vi "add.test.vi"() -> ()   [LabVIEW 2016]
uses:
  <vilib>/addons/_JKI Toolkits/Caraya/classes/Assert/Assert Equal Value_Variant.vi
  <vilib>/addons/_JKI Toolkits/Caraya/classes/Test/Test.lvclass
  <vilib>/addons/_JKI Toolkits/Caraya/classes/Assert/Assert.lvclass
panel:
  out "error out":errorcluster
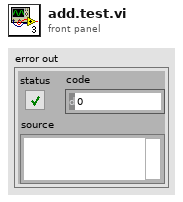
[diagram p1: front panel]
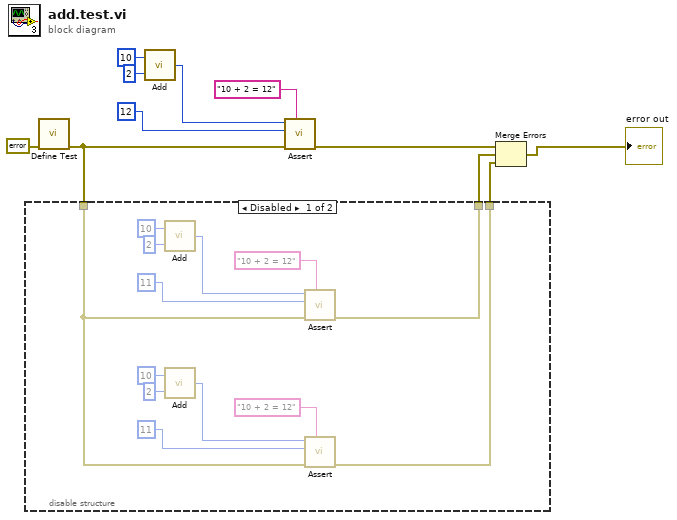
[diagram p0: block diagram]
diagram:
  n1 = call <vilib>:"Define Test.vi"("error in (no error)"=errorcluster {"status"=FALSE, "code"=0, "source"=""}) -> ("error out"=w2:errorcluster)  [unwired: 10 in]
  n2 = disable-structure shown="Disabled" {
    disable-tunnel: [w14 _] -> w3
    disable-tunnel: w2 -> [w13 _]
    disable-tunnel: [w12 _] -> w1
    frame Disabled {
      n3 = call "Add.vi"("y"=2, "x"=10) -> ("x+y"=w23:i32)
      n4 = call "Add.vi"("y"=2, "x"=10) -> ("x+y"=w16:i32)
      n5 = call-poly <vilib>:"Assert.vi"("Label"="10 + 2 = 12" ("Label (VI Title)"), "error in (no error)"=w13, "Y"=11 ("y"), "X"=w23) -> ("error out"=w14:errorcluster)  [unwired: 7 in]
      n6 = call-poly <vilib>:"Assert.vi"("Label"="10 + 2 = 12" ("Label (VI Title)"), "error in (no error)"=w13, "Y"=11 ("y"), "X"=w16) -> ("error out"=w12:errorcluster)  [unwired: 7 in]
    }
    frame Enabled {
    }
  }
  n7 = call "Add.vi"("y"=2, "x"=10) -> ("x+y"=w7:i32)
  n8 = call-poly <vilib>:"Assert.vi"("Label"="10 + 2 = 12" ("Label (VI Title)"), "error in (no error)"=w2, "Y"=12 ("y"), "X"=w7) -> ("error out"=w10:errorcluster)  [unwired: 7 in]
  n9 = Merge Errors(w10, w3, w1) -> (→"error out":errorcluster)
